vi "test_interp8.vi"() -> ()   [LabVIEW 2013]
panel:
  out "Array":fxp<+/-,16,14>[][](array[numeric])
  out "size(s)":i32
  out "Waveform Graph 3":dbl[][](graph)
  out "Waveform Graph 2":i16[](graph)
  out "Waveform Graph":dbl[](graph)
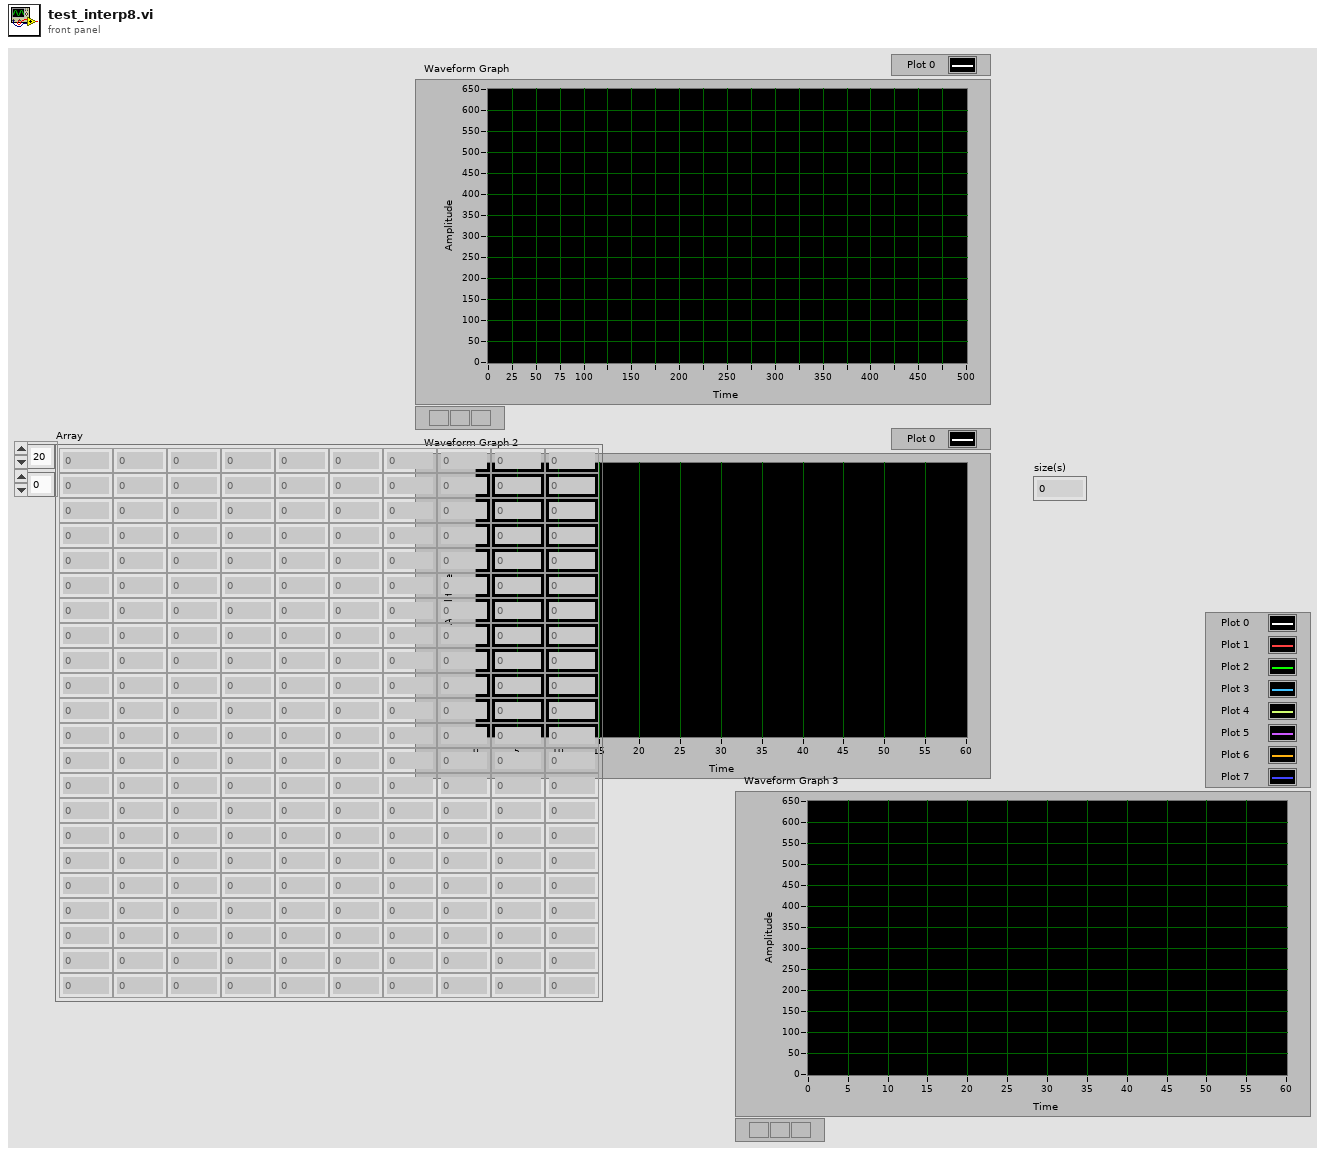
[diagram p1: front panel]
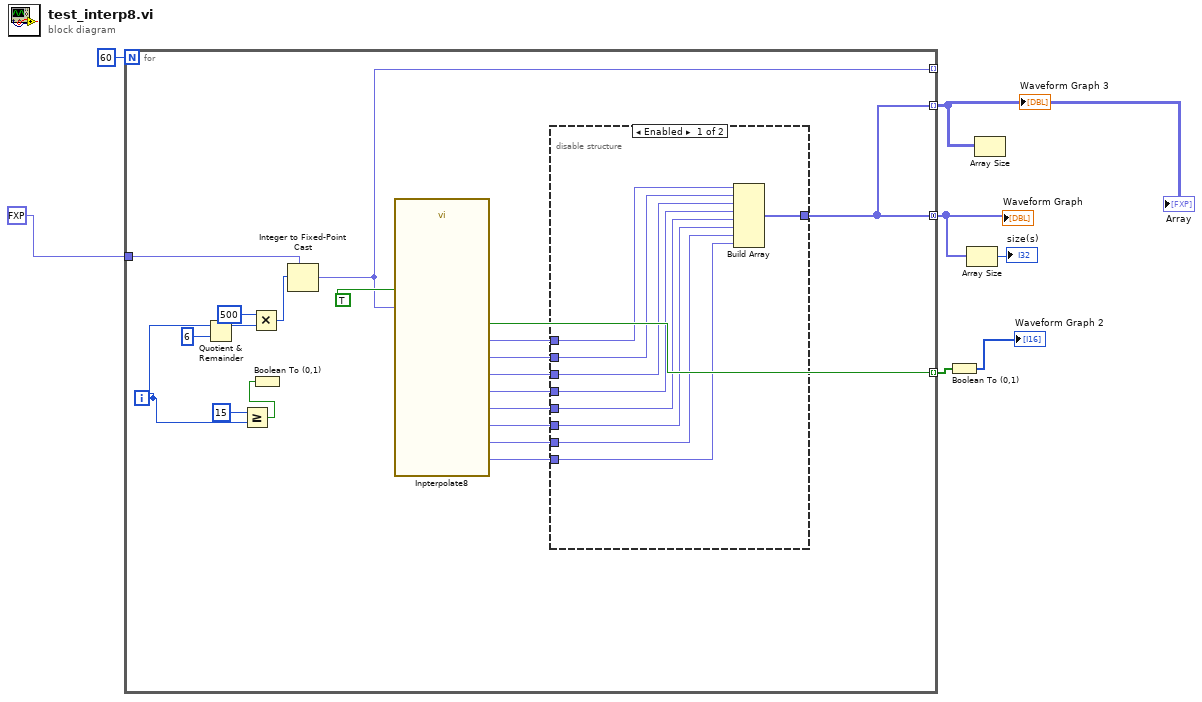
[diagram p0: block diagram]
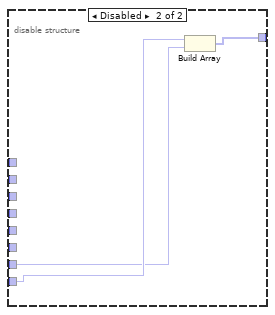
[diagram p2: hidden frame]
diagram:
  n1 = for {
    N: 60 -> [_]
    tunnel: fxp<+/-,16,14> 0.0 ("X") -> [w26]
    tunnel: [w23] -> w5 mode=indexing
    tunnel: [w9] -> w3 mode=concatenating
    tunnel: [w9] -> w1 mode=indexing
    tunnel: [w18] -> _ mode=indexing
    i -> [w22]
    n2 = Quotient & Remainder(x=w22, y=6) -> (x-y*floor(x/y)=w8:i32)  [unwired: 1 out]
    n3 = Greater Or Equal?(x=15, y=w22) -> (x >= y?=w20:bool)
    n4 = Multiply(x=500, y=w8) -> (x*y=w19:i32)
    n5 = Boolean To (0,1)(Boolean=w20) -> ()  [unwired: 1 out]
    n6 = Integer to Fixed-Point Cast(fixed-point type=w26, integer=w19) -> (fixed-point=w18:fxp<+/-,16,14>)
    n7 = call "Inpterpolate8.vi"("X"=w18, "input valid"=TRUE) -> ("X(t -7)"=w10:fxp<+/-,16,14>, "X(t -5)"=w12:fxp<+/-,16,14>, "X(t)"=w17:fxp<+/-,16,14>, "X(t -1)"=w16:fxp<+/-,16,14>, "X(t -2)"=w15:fxp<+/-,16,14>, "X(t -3)"=w14:fxp<+/-,16,14>, "X(t -6)"=w11:fxp<+/-,16,14>, "X(t -4)"=w13:fxp<+/-,16,14>, "output valid"=w23:bool)  [unwired: 5 in]
    n8 = disable-structure shown="Enabled" {
      disable-tunnel: w17 -> [w28 w39]
      disable-tunnel: w16 -> [w29 w38]
      disable-tunnel: w15 -> [w30 _]
      disable-tunnel: w14 -> [w31 _]
      disable-tunnel: w13 -> [w32 _]
      disable-tunnel: w12 -> [w33 _]
      disable-tunnel: w11 -> [w34 _]
      disable-tunnel: w10 -> [w35 _]
      disable-tunnel: [w36 w37] -> w9
      frame Enabled {
        n9 = Build Array(w35, w34, w33, w32, w31, w30, w29, w28) -> (w36:fxp<+/-,16,14>[])
      }
      frame Disabled {
        n10 = Build Array(w39, w38) -> (w37:fxp<+/-,16,14>[])
      }
    }
  }
  "Waveform Graph" <- w3
  "Waveform Graph 3" <- w1
  "Array" <- w1
  n11 = Boolean To (0,1)(Boolean=w5) -> (0, 1=→"Waveform Graph 2":i16[])
  n12 = Array Size(array=w3) -> (size(s)=→"size(s)":i32)
  n13 = Array Size(array=w1) -> ()  [unwired: 1 out]
